vi "Smart IO Get Device Channels.vi"(8 "error in (no error)":errorcluster) -> (0 "error out":errorcluster, 3 "device count":i32)   [LabVIEW 2026, in "MrcLib.lvlib"]
doc: "Returns the number of smart I/O devices that are connected to the current controller."
uses:
  MrcLib.lvlib
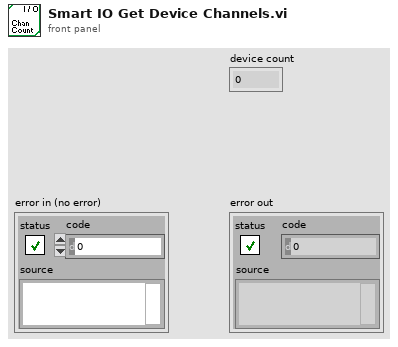
[diagram p1: front panel]
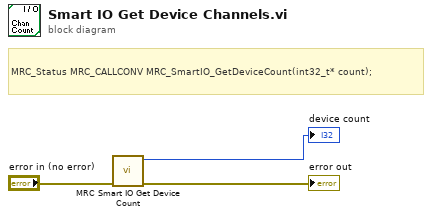
[diagram p0: block diagram]
diagram:
  # "MRC_Status MRC_CALLCONV MRC_SmartIO_GetDeviceCount(int32_t* count);"
  n1 = call "MRC Smart IO Get Device Count.vi"("error in (no error)"="error in (no error)") -> ("error out"=→"error out":errorcluster, "count out"=→"device count":i32)  [unwired: 9 in]
